vi "CheckAddsOnDeploy.vi"(5 "System Definition Dir":path, 6 "IP address":string, 7 "Details Ref":refnum<vi>, 8 "error in (no error)":errorcluster, 10 "ftp session":T2, 11 "Device Item Ref in":T1 format="%.0x") -> (0 "error out":errorcluster, 2 "ftp session out":T2, 3 "Device Item Ref out":T1 format="%.0x")   [LabVIEW 2020, in "RefMem DMA System Explorer.lvlib"]
uses:
  RefMem DMA System Explorer.lvlib
  <vilib>/FTP/ftp0.llb/FTP Session.ctl
  <vilib>/NI VeriStand/Custom Device API/Custom Device Item Ref.ctl
  <vilib>/NI VeriStand/Custom Device API/Custom Device API.lvlib
  NationalInstruments.VeriStand.SystemStorage
  Shared/Constants.vi
  Shared/RefMem DMA Shared.lvlib
  <vilib>/FTP/NI_FTP.lvlib
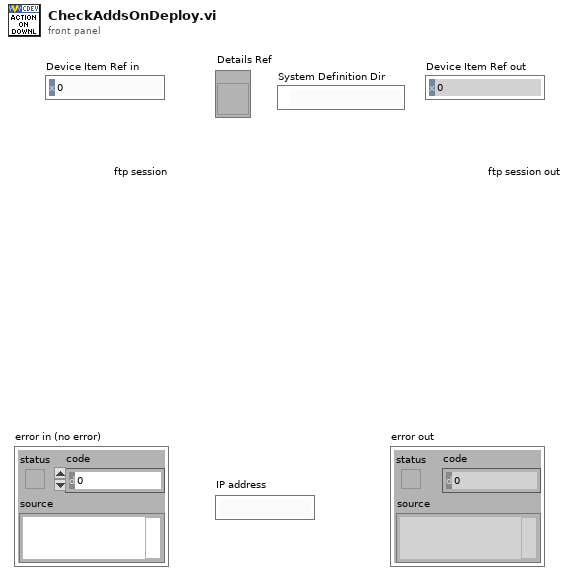
[diagram p1: front panel]
types:
  T1 = typedef "Custom Device API.lvlib/Custom Device Item Ref.ctl" = u64
  T2 = typedef "NI_FTP.lvlib/FTP Session.ctl" = refnum<k5>
  T3 = typedef "Custom Device API.lvlib/Custom Device Pointer.ctl" = refnum<k24>
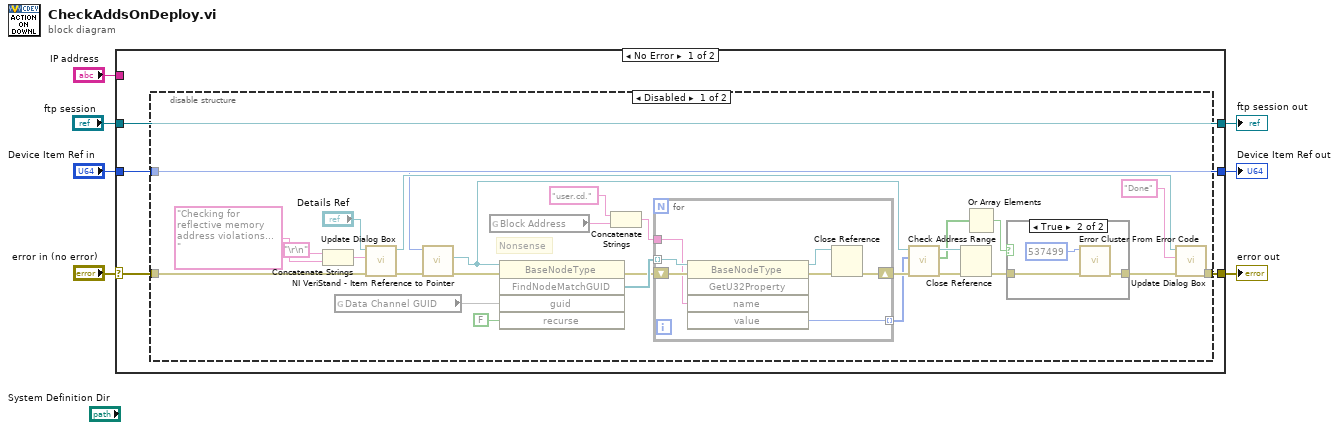
[diagram p0: block diagram]
diagram:
  n1 = case shown="No Error" "error in (no error)" {
    selector: "error in (no error)" -> [w8 w53]
    tunnel: [w10 w53] -> w6
    tunnel: "ftp session" -> [w11 w52]
    tunnel: [w11 w52] -> w4
    tunnel: "Device Item Ref in" -> [w9 w51]
    tunnel: [w9 w51] -> w2
    tunnel: "IP address" -> [_ _]
    frame No Error {
      n2 = disable-structure shown="Disabled" {
        disable-tunnel: [w35 w50] -> w10
        disable-tunnel: w9 -> [w31 _]
        disable-tunnel: w8 -> [w21 w50]
        frame Disabled {
          # "Nonsense"
          n3 = Concatenate Strings("\r\n", "Checking for reflective memory address violations... " ("string")) -> (w36:string)
          n4 = global read "Constants.vi" "Data Channel GUID"() -> (w28)
          n5 = call "Update Dialog Box.vi"("error in (no error)"=w21, "Text to add"=w36, "Details Ref in"="Details Ref") -> ("error out"=w22:errorcluster, "Details Ref out"=w34:refnum<vi>)  [unwired: 7 in]
          n6 = call <vilib>:"NI VeriStand - Item Reference to Pointer.vi"("error in (no error)"=w22, "Item Ref in"=w31) -> ("error out"=w30:errorcluster, "Node Pointer"=w18:T3)  [unwired: 6 in, 2 out]
          n7 = global read "Constants.vi" "Block Address"() -> (w25:string)
          n8 = invoke class="BaseNodeType" method="FindNodeMatchGUID"(reference=w18, error in=w30, "guid"=w28, "recurse"=FALSE) -> (error out=w26:errorcluster, "FindNodeMatchGUID"=w27:refnum<k24>[])  [unwired: 1 in, 3 out]
          n9 = Concatenate Strings("user.cd." ("string"), w25) -> (w23:string)
          n10 = for {
            tunnel: w27 -> [w48] mode=indexing
            shift-right: [w45] -> w19
            shift-left: w26 -> [w49]
            tunnel: w23 -> [w47]
            tunnel: [w43] -> w17 mode=indexing
            n11 = invoke class="BaseNodeType" method="GetU32Property"(reference=w48, error in=w49, "name"=w47) -> (reference out=w44:refnum<k24>, error out=w46:errorcluster, "value"=w43:u32)  [unwired: 2 in, 2 out]
            n12 = Close Reference(reference=w44, error in (no error)=w46) -> (error out=w45:errorcluster)
          }
          n13 = call "Check Address Range.vi"("error in (no error)"=w19, "Addresses"=w17, "Node Pointer In"=w18) -> ("error out"=w16:errorcluster, "Inside NIVS Range"=w13:bool[], "Node Pointer dup"=w14:T3)  [unwired: 6 in]
          n14 = Close Reference(reference=w14, error in (no error)=w16) -> (error out=w15:errorcluster)
          n15 = Or Array Elements(Boolean array=w13) -> (logical OR=w12:bool)
          n16 = case shown="True" w12 {
            tunnel: w15 -> [w39 w41]
            tunnel: [w39 w40] -> w20
            frame False {
            }
            frame True {
              n17 = call <vilib>:"Error Cluster From Error Code.vi"("error in (no error)"=w41, "error code (0)"=537499) -> ("error out"=w40:errorcluster)  [unwired: 7 in]
            }
          }
          n18 = call "Update Dialog Box.vi"("error in (no error)"=w20, "Text to add"="Done" ("string"), "Details Ref in"=w34) -> ("error out"=w35:errorcluster)  [unwired: 7 in, 1 out]
        }
        frame Enabled {
        }
      }
    }
    frame Error {
    }
  }
  "error out" <- w6
  "ftp session out" <- w4
  "Device Item Ref out" <- w2
